vi "Retrive Data.vi"(8 "error in (no error)":errorcluster, 9 "Tag":string, 10 "Tree In":refnum<class "Tree.lvclass">, 11 "Composite Tree Data in":refnum<class "Composite Tree Data.lvclass">) -> (0 "error out":errorcluster, 1 "Data Out":T1, 2 "Tree Out":refnum<class "Tree.lvclass">, 3 "Composite Tree Data out":refnum<class "Composite Tree Data.lvclass">, 5 "Data Group Out":T1[](array[typedef]))   [LabVIEW 2022 SP3, in "Composite Tree Data.lvclass"]
uses:
  Composite Tree Data.lvclass
  Tree/Tree.lvclass
  Tree/Type Def/Tree Item.ctl
  Composite Tree Data.lvclass/Composite Tree Data.ctl
  Tree Data/Tree Data.lvclass
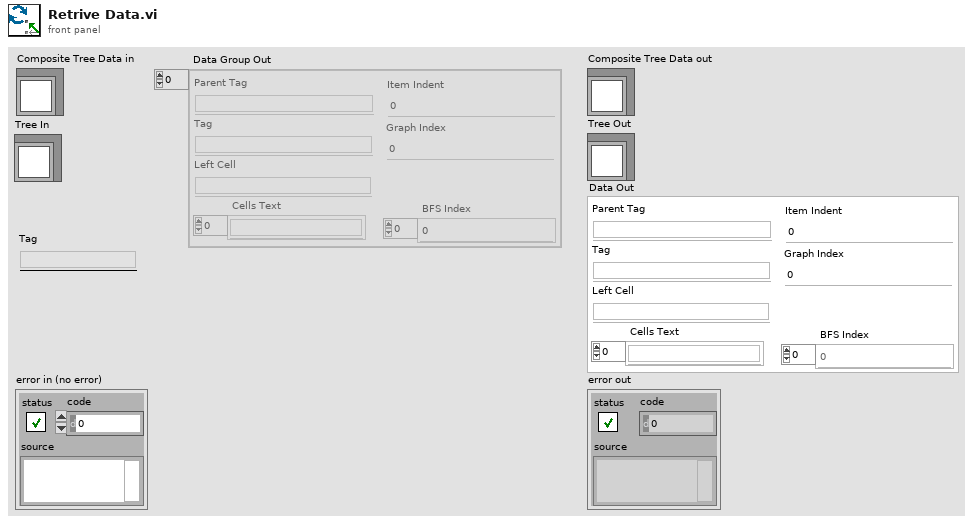
[diagram p1: front panel]
types:
  T1 = typedef "Tree Item.ctl" = cluster{"Parent Tag":string, "Tag":string, "Left Cell":string, "Cells Text":string[], "BFS Index":i32[], "Graph Index":i32, "Item Indent":i32}
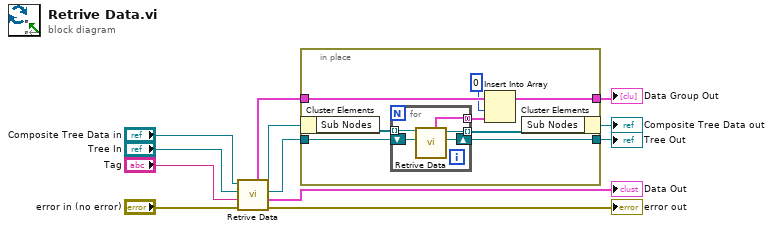
[diagram p0: block diagram]
diagram:
  n1 = call-parent "Retrive Data.vi"("error in (no error)"="error in (no error)", "Tag"="Tag", "Tree In"="Tree In", "Tree Data in"="Composite Tree Data in") -> ("error out"=→"error out":errorcluster, "Data Out"=→"Data Out":T1, "Tree Out"=w4:refnum<class "Tree.lvclass">, "Tree Data out"=w6:refnum<class "Composite Tree Data.lvclass">, "Data Group Out"=w5:T1[])  [unwired: 3 in]
  n2 = in-place {
    in-place-border: w5 -> [w16]
    in-place-border: w4 -> [w18]
    in-place-border: [w17] -> w2
    in-place-border: [w13] -> w1
    n3 = in-place-cluster #1(w6) -> ("Sub Nodes"=w20:refnum<class "Tree Data.lvclass">[])
    n4 = for {
      tunnel: w20 -> [w25] mode=indexing
      tunnel: [w24] -> w19 mode=indexing
      shift-right: [w22] -> w17
      shift-left: w18 -> [w23]
      tunnel: [w21] -> w15 mode=concatenating
      n5 = call-dynamic "Retrive Data.vi"("Tree In"=w23, "Tree Data in"=w25) -> ("Tree Out"=w22:refnum<class "Tree.lvclass">, "Tree Data out"=w24:refnum<class "Tree Data.lvclass">, "Data Group Out"=w21:T1[])  [unwired: 5 in, 2 out]
    }
    n6 = Insert Into Array(array=w16, index=0, new element=w15) -> (w13:T1[])
    n7 = in-place-cluster #1("Sub Nodes"=w19) -> (→"Composite Tree Data out":refnum<class "Composite Tree Data.lvclass">)
  }
  "Tree Out" <- w2
  "Data Group Out" <- w1
